vi "Map to Local Path.vi"(7 "Use base-path? (T)":bool=TRUE, 8 "error in (no error)":errorcluster, 9 "Query":variant, 10 "Local Path":path, 11 "URI in":refnum<class "URI.lvclass">) -> (0 "error out":errorcluster, 1 "Appended Query":variant, 2 "Mapped Local Path":path, 3 "URI out":refnum<class "URI.lvclass">)   [LabVIEW 2013, in "openURI.lvlib" / "URI.lvclass"]
uses:
  URI.lvclass
  URI.lvclass/URI.ctl
  components/path/Get path (absolute).vi
  components/path/Get path (relative-base).vi
  openURI.lvlib
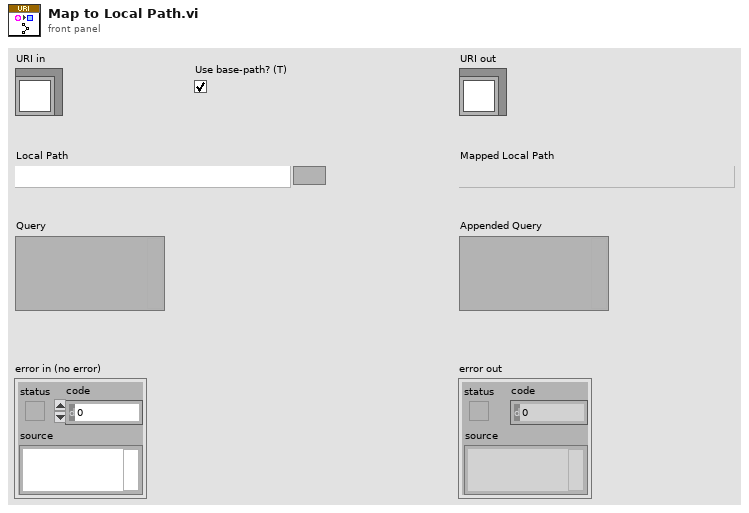
[diagram p1: front panel]
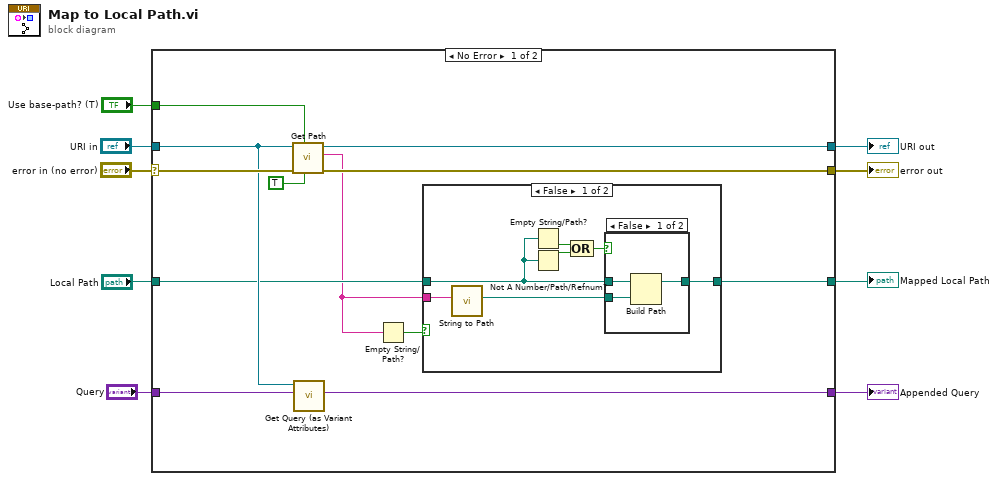
[diagram p0: block diagram]
diagram:
  n1 = case shown="No Error" "error in (no error)" {
    selector: "error in (no error)" -> [w20 w37]
    tunnel: [w19 w37] -> w8
    tunnel: [w21 w36] -> w6
    tunnel: "URI in" -> [w16 w36]
    tunnel: "Local Path" -> [w13 w35]
    tunnel: [w17 w35] -> w4
    tunnel: [w15 w34] -> w3
    tunnel: "Query" -> [w14 w34]
    tunnel: "Use base-path? (T)" -> [w10 _]
    frame No Error {
      n2 = call "Get Path.vi"("Strip lead \"/\" (F)"=TRUE ("Strip lead \"/\" (F)"), "Use base-path?"=w10, "error in (no error)"=w20, "URI in"=w16) -> ("error out"=w19:errorcluster, "path"=w11:string, "URI out"=w21:refnum<class "URI.lvclass">)  [unwired: 5 in]
      n3 = call "Get Query (as Variant Attributes).vi"("Container (default: new variant)"=w14, "URI in"=w16) -> ("Container with Query Attributes"=w15:variant)  [unwired: 7 in, 2 out]
      n4 = Empty String/Path?(string/path=w11) -> (empty?=w12:bool)
      n5 = case shown="False" w12 {
        tunnel: [w28 w33] -> w17
        tunnel: w13 -> [w26 w33]
        tunnel: w11 -> [w25 _]
        frame False {
          n6 = call "String to Path.vi"("common path"=w25) -> ("Path"=w27:path)  [unwired: 10 in]
          n7 = Empty String/Path?(string/path=w26) -> (empty?=w24:bool)
          n8 = Not A Number/Path/Refnum?(number/path/refnum=w26) -> (NaN/Path/Refnum?=w23:bool)
          n9 = Compound Arithmetic op=OR(w24, w23) -> (w22:bool)
          n10 = case shown="False" w22 {
            tunnel: [w31 w32] -> w28
            tunnel: w27 -> [w30 w32]
            tunnel: w26 -> [w29 _]
            frame False {
              n11 = Build Path(base path=w29, name or relative path=w30) -> (appended path=w31:path)
            }
            frame True {
            }
          }
        }
        frame True {
        }
      }
    }
    frame Error {
    }
  }
  "error out" <- w8
  "URI out" <- w6
  "Mapped Local Path" <- w4
  "Appended Query" <- w3
